vi "AI-Volt-Clock.vi"(6 "Slot":T1, 8 "error in":errorcluster, 10 "Mode":string, 11 "CH":string) -> (0 "error out":errorcluster, 3 "data":dbl caption="数据" format="%0.2f")   [LabVIEW 2013]
uses:
  SystemCode/SysControl/Slot.ctl
  <vilib>/DAQmx/read.llb/DAQmx Read (Analog Wfm 1Chan NSamp).vi
  SourceCode/GlobalValue.vi
  <vilib>/DAQmx/create/channels.llb/DAQmx Create Channel (AI-Voltage-Basic).vi
  <vilib>/DAQmx/configure/timing.llb/DAQmx Timing (Sample Clock).vi
  <vilib>/measure/madcrms.llb/Basic Averaged DC-RMS for 1 Chan.vi
  <vilib>/DAQmx/miscellaneous.llb/DAQmx Fill In Error Info.vi
  <vilib>/measure/NI_MAPro.lvlib
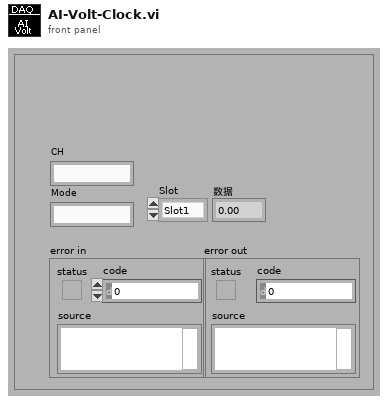
[diagram p1: front panel]
types:
  T1 = typedef "Slot.ctl" = enum16{"Slot1", "Slot2", "Slot3", "Slot4"}
  T2 = typedef "DAQConfig.ctl" = cluster{"DIO":string[][], "AO":string[][], "AI":string[][]}
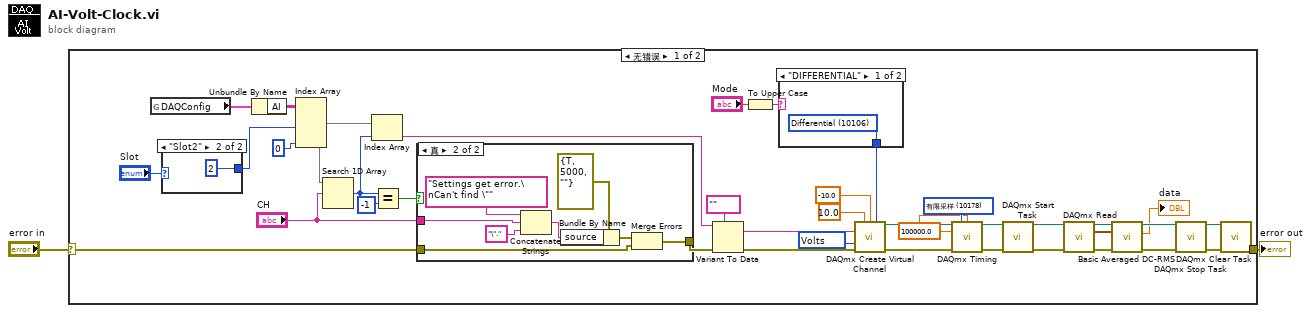
[diagram p0: block diagram]
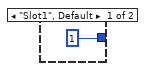
[diagram p2: hidden frame]
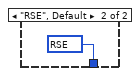
[diagram p3: hidden frame]
diagram:
  n1 = case shown="无错误" "error in" {
    selector: "error in" -> [w21 w55]
    tunnel: [w41 w55] -> w2
    frame No Error {
      w5 = 100000.0 ("rate")
      w16 = 10178 items=["有限采样"=10178, "连续采样"=10123, "硬件定时单点"=12522] ("sample mode")
      w37 = 10348 items=["Volts"=10348, "From Custom Scale"=10065] ("units")
      n2 = global read "GlobalValue.vi" "DAQConfig"() -> (w3:T2)
      n3 = case shown="\"Slot2\"" "Slot" {
        tunnel: [1 ("索引 (行)") 2 ("索引 (行)")] -> w6
        frame "Slot1", Default {
        }
        frame "Slot2" {
        }
      }
      n4 = Unbundle By Name(w3) -> ("AI"=w33:string[][])
      n5 = Index Array(array=w33, index (col) #1=w6, index (col) #2=0 ("索引 (列)")) -> (element #1=w29:string[], element #2=w28:string[])  [unwired: 2 in]
      n6 = Search 1D Array(1D array=w28, element="CH") -> (index of element=w31:i32)  [unwired: 1 in]
      n7 = Index Array(array=w29, index=w31) -> (element=w20:string)
      n8 = Equal?(x=w31, y=-1) -> (x = y?=w27:bool)
      n9 = case shown="真" w27 {
        tunnel: w21 -> [w46 w50]
        tunnel: [w46 w49] -> w22
        tunnel: "CH" -> [_ w48]
        frame False {
        }
        frame True {
          n10 = Concatenate Strings("Settings get error.\nCan't find \"" ("message"), w48, "\"." ("string")) -> (w53:string)
          n11 = Bundle By Name(cluster=errorcluster {"status"=TRUE, "code"=5000, "source"=""} ("error in 1 (no error)"), "source"=w53) -> (w52:errorcluster)
          n12 = Merge Errors(w52, w50) -> (w49:errorcluster)
        }
      }
      n13 = Variant To Data(error in=w22, type=tag "" ("lines"), Variant=w20) -> (data=w24:tag, error out=w23:errorcluster)
      n14 = To Upper Case(1:"Mode") -> (0:w18:string)
      n15 = case shown="\"DIFFERENTIAL\"" w18 {
        tunnel: [w44 w45] -> w17
        frame "DIFFERENTIAL" {
          w44 = 10106 items=["default"=-1, "RSE"=10083, "NRSE"=10078, "Differential"=10106, "Pseudodifferential"=12529] ("input terminal configuration")
        }
        frame "RSE", Default {
          w45 = 10083 items=["default"=-1, "RSE"=10083, "NRSE"=10078, "Differential"=10106, "Pseudodifferential"=12529] ("input terminal configuration")
        }
      }
      n16 = call-poly <vilib>:"DAQmx Create Virtual Channel.vi"("maximum value"=10.0, "minimum value"=-10.0, "input terminal configuration"=w17, "physical channels"=w24, "units"=w37, "error in"=w23) -> ("task out"=w15:refnum<k21>, "error out"=w13:errorcluster)  [unwired: 8 in]
      n17 = call-poly <vilib>:"DAQmx Timing.vi"("task/channels in"=w15, "sample mode"=w16, "samples per channel"=w5, "rate"=w5, "error in"=w13) -> ("task out"=w14:refnum<k21>, "error out"=w12:errorcluster)  [unwired: 2 in, 7 out]
      n18 = call <vilib>:"DAQmx Start Task.vi"("task/channels in"=w14, "error in"=w12) -> ("task out"=w4:refnum<k21>, "error out"=w40:errorcluster)  [unwired: 12 in]
      n19 = call-poly <vilib>:"DAQmx Read.vi"("task/channels in"=w4, "error in"=w40) -> ("task out"=w36:refnum<k21>, "data"=w11:waveform(dbl), "error out"=w10:errorcluster)  [unwired: 11 in]
      n20 = call-poly <vilib>:"Basic Averaged DC-RMS.vi"("error in (no error)"=w10, "signal in"=w11) -> ("error out"=w9:errorcluster, "RMS value"=→"data":dbl)  [unwired: 6 in, 2 out]
      n21 = call <vilib>:"DAQmx Stop Task.vi"("task/channels in"=w36, "error in"=w9) -> ("task out"=w39:refnum<k21>, "error out"=w38:errorcluster)  [unwired: 12 in]
      n22 = call <vilib>:"DAQmx Clear Task.vi"("task in"=w39, "error in"=w38) -> ("error out"=w41:errorcluster)  [unwired: 13 in]
    }
    frame Error {
    }
  }
  "error out" <- w2
